vi "Тест_буфера.vi"() -> ()   [LabVIEW 2017]
panel:
  out "appended array 2":dbl[][](array[numeric])
  in  "Размер окна":i32=4
  out "size(s)":i32[](array[numeric])
  out "Выход последовательного массива":dbl[](array[numeric])
  in  "Последовательный массив":i32=16
  out "Array":dbl[][](array[numeric])
  in  "Размер окна буффера":i32
  out "Количество бит":i32
  in  "Количество бит":i32=8
  out "Биты на выходе":dbl[](array[numeric])
  # "3"
  # "15"
  # "7"
  # "3"
  # "7"
  # "15"
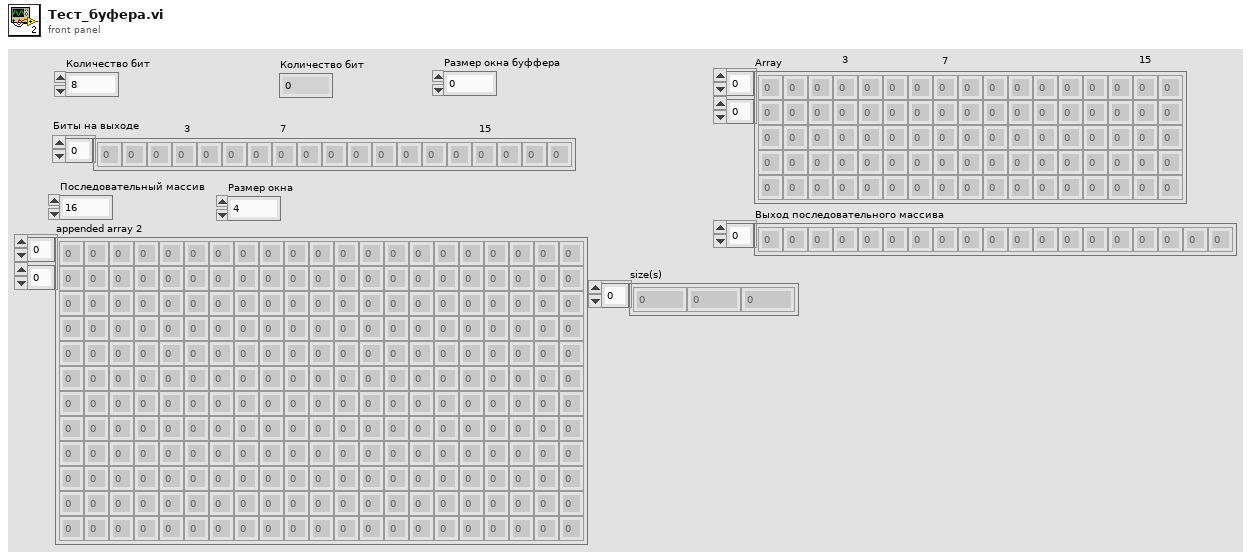
[diagram p1: front panel]
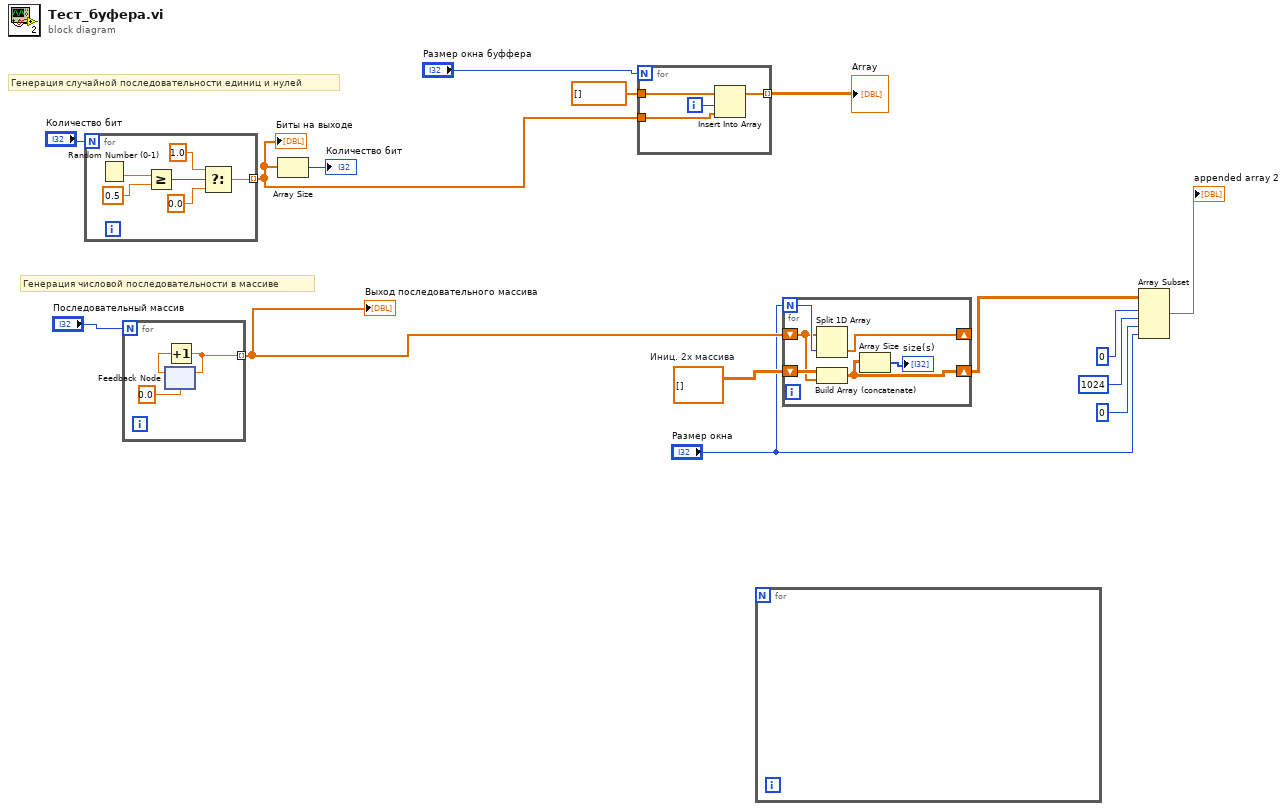
[diagram p0: block diagram]
diagram:
  w8 = dbl[][] []  # Иниц. 2х массива
  # "Генерация числовой последовательности в массиве"
  # "Генерация случайной последовательности единиц и нулей"
  n1 = for {
    N: "Количество бит" -> [_]
    tunnel: [w16] -> w10 mode=indexing
    n2 = Random Number (0-1)() -> (number: 0 to 1=w21:dbl)
    n3 = Greater Or Equal?(x=w21, y=0.5) -> (x >= y?=w19:bool)
    n4 = Select(t=1.0, s=w19, f=0.0) -> (s? t:f=w16:dbl)
  }
  "Биты на выходе" <- w10
  n5 = for {
    N: "Последовательный массив" -> [_]
    tunnel: [w22] -> w7 mode=indexing
    n6 = feedback #1(0.0) -> (w24:dbl)
    n7 = Increment(x=w24) -> (x+1=w22:dbl)
    n8 = feedback-in #1(w22) -> ()
  }
  "Выход последовательного массива" <- w7
  n9 = Array Size(array=w10) -> (size(s)=→"Количество бит":i32)
  n10 = for {
    N: "Размер окна буффера" -> [_]
    tunnel: w10 -> [w26]
    tunnel: dbl[] [] -> [w27]
    tunnel: [w28] -> w13 mode=indexing
    i -> [w25]
    n11 = Insert Into Array(array=w27, index=w25, new element=w26) -> (w28:dbl[])
  }
  "Array" <- w13
  n12 = for {
  }
  n13 = for {
    N: "Размер окна" -> [w31]
    shift-right: [w33] -> w6
    shift-left: w8 -> [w34]
    shift-right: [w30] -> _
    shift-left: w7 -> [w29]
    n14 = Split 1D Array(array=w29, index=w31) -> (second subarray=w30:dbl[])  [unwired: 1 out]
    n15 = Build Array (concatenate)(w34, w29) -> (w33:dbl[][])
    n16 = Array Size(array=w33) -> (size(s)=→"size(s)":i32[])
  }
  n17 = Array Subset(array=w6, index (row)=0 ("length"), length (row)=1024 ("length"), index (col)=0 ("index"), length (col)="Размер окна") -> (→"appended array 2":dbl[][])
